vi "Configure Apply DPD Crest Factor Reduction.vi"(0 "Instrument Handle In":refnum<k21>, 1 "Selector String":string, 5 "Apply DPD Crest Factor Reduction Configuration":T1={"Enabled"=1, "Method"=0, "Max Iterations"=10, "Target PAPR Type"=0, "Target PAPR (dB)"=8.0, "Window Type"=7, "Window Length"=10, "Shaping Factor"=5.0, "Shaping Threshold (dB)"=-5.0} {"Target PAPR Type" items=["Input PAPR", "Custom"]; "Window Type" items=["Flat Top"=1, "Hanning"=2, "Hamming"=3, "Gaussian"=4, "Blackman"=5, "Blackman-Harris"=6, "Kaiser-Bessel"=7]; "Method" items=["Clipping", "Peak Windowing", "Sigmoid"]; "Enabled" items=["False", "True"]}, 11 "error in (no error)":errorcluster) -> (4 "Instrument Handle Out":refnum<k21>, 15 "error out":errorcluster)   [LabVIEW 2016, in "RFmxDPD.lvlib"]
uses:
  RFmxDPD.lvlib
  Typedefs/Apply DPD Crest Factor Reduction Configuration.ctl
  <resource>/objmgr/RFmxSpecAn.rc
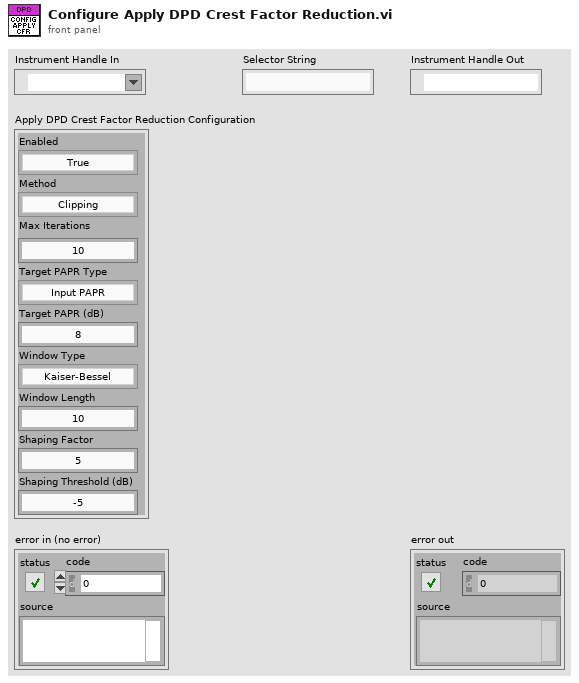
[diagram p1: front panel]
types:
  T1 = typedef "RFmxDPD.lvlib/Apply DPD Crest Factor Reduction Configuration.ctl" = cluster{"Enabled":i32, "Method":i32, "Max Iterations":i32, "Target PAPR Type":i32, "Target PAPR (dB)":dbl, "Window Type":i32, "Window Length":i32, "Shaping Factor":dbl, "Shaping Threshold (dB)":dbl}
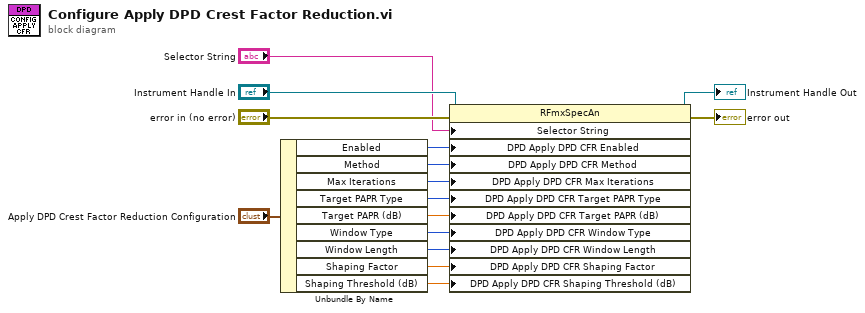
[diagram p0: block diagram]
diagram:
  n1 = Unbundle By Name("Apply DPD Crest Factor Reduction Configuration") -> ("Enabled"=w1:i32, "Method"=w9:i32, "Max Iterations"=w8:i32, "Target PAPR Type"=w7:i32, "Target PAPR (dB)"=w6:dbl, "Window Type"=w5:i32, "Window Length"=w4:i32, "Shaping Factor"=w3:dbl, "Shaping Threshold (dB)"=w2:dbl)
  n2 = property class="RFmxSpecAn"(reference="Instrument Handle In", error in="error in (no error)", "Selector String"="Selector String", "DPD Apply DPD CFR Enabled"=w1, "DPD Apply DPD CFR Method"=w9, "DPD Apply DPD CFR Max Iterations"=w8, "DPD Apply DPD CFR Target PAPR Type"=w7, "DPD Apply DPD CFR Target PAPR (dB)"=w6, "DPD Apply DPD CFR Window Type"=w5, "DPD Apply DPD CFR Window Length"=w4, "DPD Apply DPD CFR Shaping Factor"=w3, "DPD Apply DPD CFR Shaping Threshold (dB)"=w2) -> (reference out=→"Instrument Handle Out":refnum<k21>, error out=→"error out":errorcluster)
